vi "dvp Vi Set Black Level.vi"(10 "BlackLevel":sgl, 11 "handle":u32) -> (3 "function return":u32(ring))   [LabVIEW 2018, in "LabViewDVPCamera.lvlib"]
doc: "LabviewDvp2Api dvpStatus dvpViSetBlackLevel(dvpHandle handle, float BlackLevel);"
uses:
  LabViewDVPCamera.lvlib
  LabViewDVPCamera/LabViewDVPCamera.dll
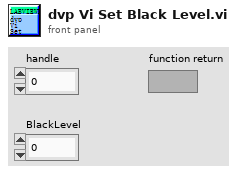
[diagram p1: front panel]
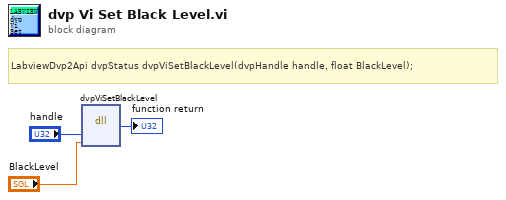
[diagram p0: block diagram]
diagram:
  # "LabviewDvp2Api dvpStatus dvpViSetBlackLevel(dvpHandle handle, float BlackLevel);"
  n1 = dll-call lib="C:/Program Files (x86)/DVP2 Labview cn 64/Sample/LabViewDVPCamera/LabViewDVPCamera.*" fn="dvpViSetBlackLevel"("handle"="handle", "BlackLevel"="BlackLevel") -> (→"function return":u32)  [unwired: 5 in, 2 out]
